vi "Save Config.vi"(9 "Path":path, 10 "Cluster 2":T1, 11 "error in (no error)":errorcluster) -> (0 "refnum out":refnum<file>, 1 "cancelled":bool, 3 "error out":errorcluster)   [LabVIEW 2026]
uses:
  ConfigCluster.ctl
  Config Clusters/Channel Setup/(Main) Channel Setup.ctl
  Config Clusters/Channel Setup/Channel Interfaces.ctl
  Config Clusters/Channel Setup/Micropulse.ctl
  Config Clusters/Channel Setup/Gates.ctl
  Config Clusters/Scan Setup/(Main) Scan Setup.ctl
  Config Clusters/Scan Setup/Scan Information.ctl
  Config Clusters/Scan Setup/Scan Settings.ctl
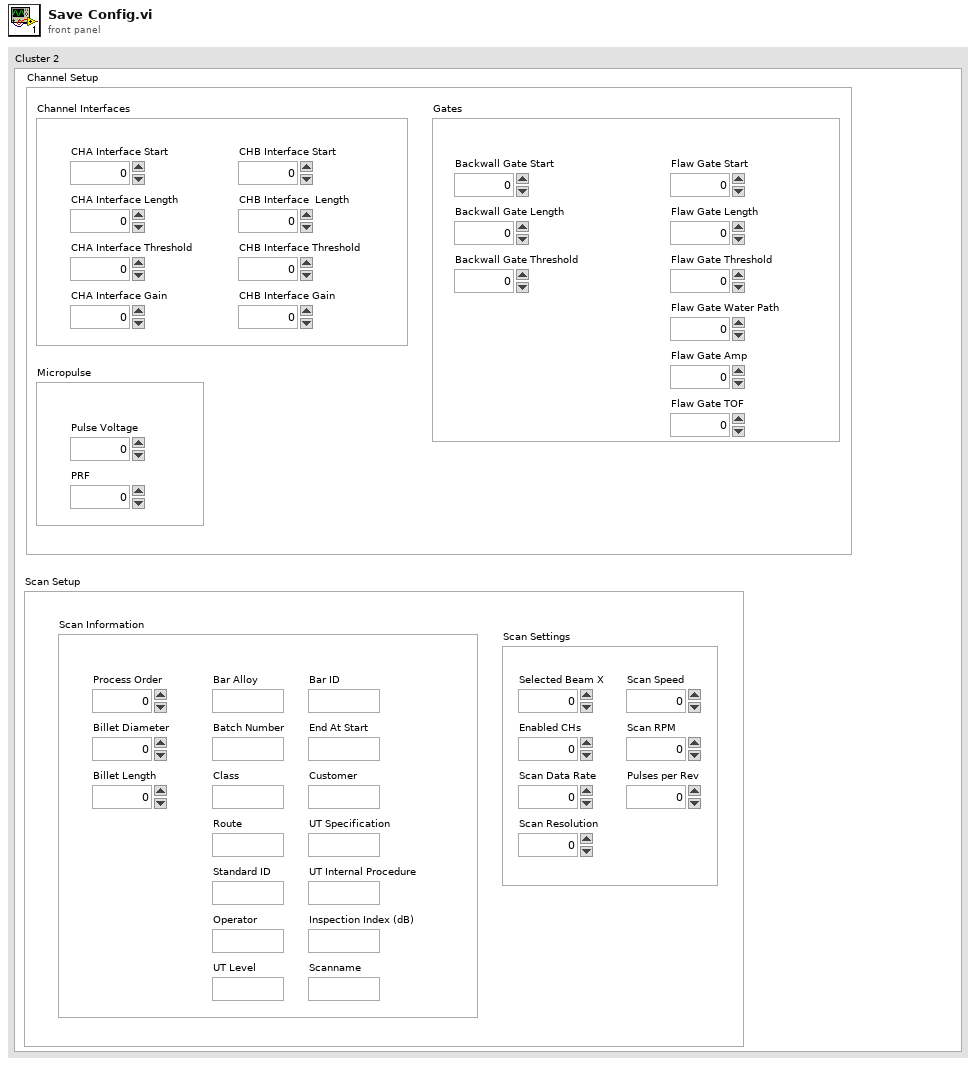
[diagram p1: front panel]
types:
  T1 = typedef "ConfigCluster.ctl" = cluster{"Channel Setup":T2, "Scan Setup":T6}
  T2 = typedef "(Main) Channel Setup.ctl" = cluster{"Channel Interfaces":T3, "Micropulse":T4, "Gates":T5}
  T3 = typedef "Channel Interfaces.ctl" = cluster{"CHA Interface Start":dbl, "CHA Interface Length":dbl, "CHA Interface Threshold":dbl, "CHA Interface Gain":dbl, "CHB Interface Start":dbl, "CHB Interface  Length ":dbl, "CHB Interface Threshold":dbl, "CHB Interface Gain":dbl}
  T4 = typedef "Micropulse.ctl" = cluster{"Pulse Voltage":dbl, "PRF":dbl}
  T5 = typedef "Gates.ctl" = cluster{"Backwall Gate Start":dbl, "Backwall Gate Length":dbl, "Backwall Gate Threshold":dbl, "Flaw Gate Start":dbl, "Flaw Gate Length":dbl, "Flaw Gate Threshold":dbl, "Flaw Gate Water Path":dbl, "Flaw Gate Amp":dbl, "Flaw Gate TOF":dbl}
  T6 = typedef "(Main) Scan Setup.ctl" = cluster{"Scan Information":T7, "Scan Settings":T8}
  T7 = typedef "Scan Information.ctl" = cluster{"Process Order":dbl, "Billet Diameter":dbl, "Billet Length":dbl, "Bar Alloy":string, "Batch Number":string, "Class":string, "Route":string, "Standard ID":string, "Bar ID":string, "End At Start":string, "Customer":string, "UT Specification":string, "UT Internal Procedure":string, "Operator":string, "UT Level":string, "Inspection Index (dB)":string, "Scanname":string}
  T8 = typedef "Scan Settings.ctl" = cluster{"Selected Beam X":dbl, "Enabled CHs":dbl, "Scan Data Rate":dbl, "Scan Resolution":dbl, "Scan Speed":dbl, "Scan RPM":dbl, "Pulses per Rev":dbl}
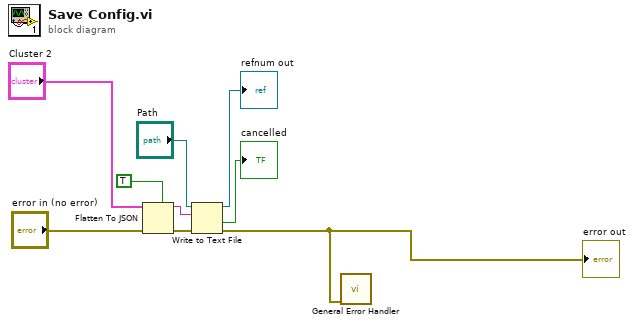
[diagram p0: block diagram]
diagram:
  n1 = Flatten To JSON(enable LabVIEW extensions? (T)=TRUE, anything="Cluster 2", error in (no error)="error in (no error)") -> (JSON string=w6:string, 11:w4:errorcluster)
  n2 = Write to Text File(file (use dialog)="Path", text=w6, error in=w4) -> (refnum out=→"refnum out":refnum<file>, cancelled=→"cancelled":bool, error out=w1:errorcluster)  [unwired: 1 in]
  "error out" <- w1
  n3 = call <vilib>:"General Error Handler.vi"("error in (no error)"=w1) -> ()  [unwired: 10 in, 5 out]
